vi "工件信息输入_子VI.vi"(8 "Y Resolution":i32, 9 "X Resolution":i32, 10 "输入的灰度阈值":dbl) -> (0 "质量等级":string, 1 "模式选择":u16(ring) items=["只读穿透图", "穿透图和反射图结合"], 2 "灰度阈值":dbl, 3 "产品规格":cluster{"产品长度（周长）（mm）":dbl, "产品宽度（母线长）（mm）":dbl}, 4 "是否需要预处理":u16, 5 "图像分辨率":T1)   [LabVIEW 2018]
panel:
  in  "是否需要预处理（默认不进行预处理）":u16(ring) items=["不需要预处理", "需要预处理"]
  in  "模式选择（默认只读穿透图）":u16(ring) items=["只读穿透图", "穿透图和反射图结合"]
  in  "质量等级（请填入A/B/C，默认为B）":u16(ring) items=["A", "B", "C"]
  in  "灰度阈值（0-255）":dbl min=0.0 max=255.0 step=1.0 format="%#_13g"
  out "错误常量out":errorcluster
  in  "错误常量":errorcluster
  in  "停止按钮":bool
  in  "产品宽度（母线长）（mm）":dbl format="%#_13g"
  in  "产品长度（周长）（mm）":dbl format="%#_13g"
  in  "图像Y向分辨率（mm/像素）":dbl=1.0 format="%#_13g"
  in  "图像X向分辨率（mm/像素）":dbl=1.0 format="%#_13g"
  # "图像及工件参数输入"
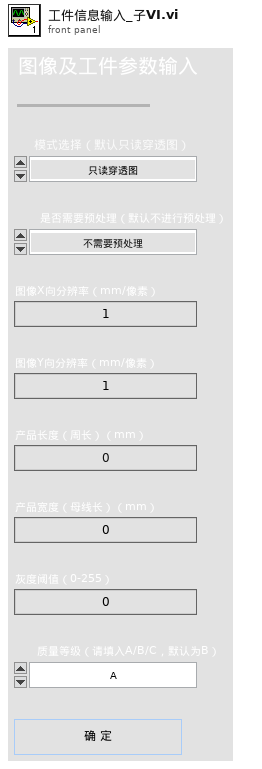
[diagram p1: front panel]
types:
  T1 = cluster{"图像X向分辨率（mm/像素）":dbl, "图像Y向分辨率（mm/像素）":dbl}
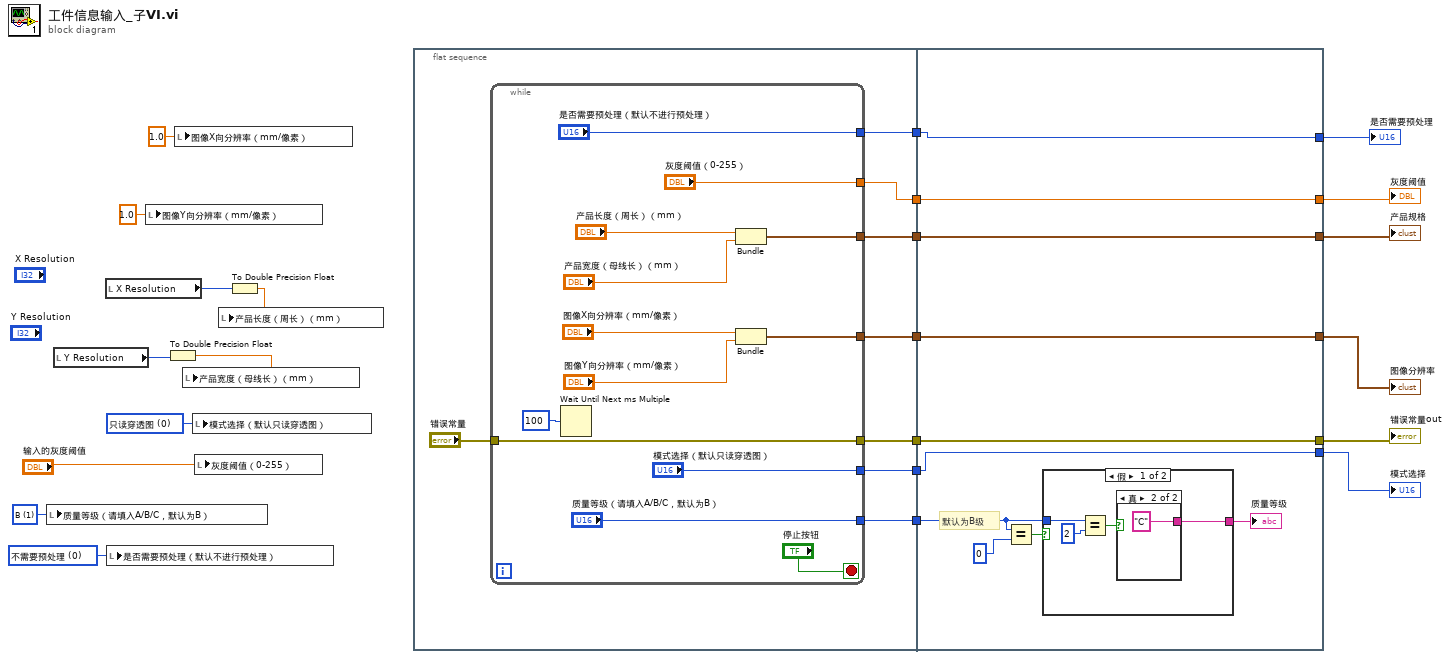
[diagram p0: block diagram]
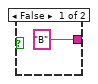
[diagram p2: hidden frame]
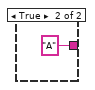
[diagram p3: hidden frame]
diagram:
  w9 = u16 0 items=["不需要预处理", "需要预处理"] ("是否需要预处理（默认不进行预处理）")
  w17 = u16 1 items=["A", "B", "C"] ("质量等级（请填入A/B/C，默认为B）")
  w18 = u16 0 items=["只读穿透图", "穿透图和反射图结合"] ("模式选择（默认只读穿透图）")
  n1 = local write "质量等级（请填入A/B/C，默认为B）"(w17) -> ()
  n2 = local read "Y Resolution"() -> (w14:i32)
  n3 = local read "X Resolution"() -> (w16:i32)
  n4 = local write "是否需要预处理（默认不进行预处理）"(w9) -> ()
  n5 = local write "图像Y向分辨率（mm/像素）"(1.0 ("图像Y向分辨率（mm/像素）")) -> ()
  n6 = To Double Precision Float(number=w14) -> (double precision float=w13:dbl)
  n7 = local write "图像X向分辨率（mm/像素）"(1.0 ("图像X向分辨率（mm/像素）")) -> ()
  n8 = local write "产品宽度（母线长）（mm）"(w13) -> ()
  n9 = local write "模式选择（默认只读穿透图）"(w18) -> ()
  n10 = local write "灰度阈值（0-255）"("输入的灰度阈值") -> ()
  n11 = To Double Precision Float(number=w16) -> (double precision float=w15:dbl)
  n12 = local write "产品长度（周长）（mm）"(w15) -> ()
  n13 = flat-sequence {
    tunnel: [w31] -> w8
    tunnel: [w30] -> w7
    tunnel: [w29] -> w6
    tunnel: [w28] -> w5
    tunnel: [w27] -> w4
    tunnel: [w26] -> w3
    tunnel: [w24] -> w2
    tunnel: [w50] -> w19
    tunnel: [w51] -> w20
    tunnel: [w52] -> w21
    tunnel: [w53] -> w22
    tunnel: [w54] -> w23
    tunnel: w8 -> [w54]
    tunnel: w7 -> [w53]
    tunnel: w6 -> [w52]
    tunnel: w5 -> [w51]
    tunnel: w4 -> [w50]
    tunnel: w3 -> [w47]
    tunnel: w2 -> [w45]
    tunnel: [w45] -> w1
    frame #0 {
      n14 = while {
        tunnel: [w44] -> w31
        tunnel: [w43] -> w30
        tunnel: "错误常量" -> [w37]
        tunnel: [w37] -> w29
        tunnel: ["灰度阈值（0-255）"] -> w28
        tunnel: ["质量等级（请填入A/B/C，默认为B）"] -> w26
        tunnel: ["模式选择（默认只读穿透图）"] -> w27
        tunnel: ["是否需要预处理（默认不进行预处理）"] -> w24
        stop <- "停止按钮" stop-if-true
        n15 = Wait Until Next ms Multiple(millisecond multiple=u32 100 ("毫秒倍数")) -> ()  [unwired: 1 out]
        n16 = Bundle("产品长度（周长）（mm）"="产品长度（周长）（mm）", "产品宽度（母线长）（mm）"="产品宽度（母线长）（mm）") -> (w43:cluster{"产品长度（周长）（mm）":dbl, "产品宽度（母线长）（mm）":dbl})  [unwired: 1 in]
        n17 = Bundle("图像X向分辨率（mm/像素）"="图像X向分辨率（mm/像素）", "图像Y向分辨率（mm/像素）"="图像Y向分辨率（mm/像素）") -> (w44:T1)  [unwired: 1 in]
      }
    }
    frame #1 {
      # "默认为B级"
      n18 = Equal?(x=w47, y=u16 0) -> (x = y?=w48:bool)
      n19 = case shown="假" w48 {
        tunnel: [w55 "A" ("质量等级")] -> w49
        tunnel: w47 -> [w57 _]
        frame False {
          n20 = Equal?(x=w57, y=u16 2) -> (x = y?=w56:bool)
          n21 = case shown="真" w56 {
            tunnel: ["B" ("质量等级") "C" ("质量等级")] -> w55
            frame False {
            }
            frame True {
            }
          }
        }
        frame True {
        }
      }
      "质量等级" <- w49
    }
  }
  "图像分辨率" <- w23
  "产品规格" <- w22
  "错误常量out" <- w21
  "灰度阈值" <- w20
  "模式选择" <- w19
  "是否需要预处理" <- w1
